vi "RegisterGUIObjectToResize.vi"(5 "Resize Object?":bool=TRUE, 8 "error in (no error)":errorcluster, 9 "Behaviour":T1 {"Adjust" items=["Height", "Width", "Both"]}, 10 "Any Control reference":refnum<vi>, 11 "PentaPanesGUI in":refnum<class "PentaPanes.lvclass">) -> (0 "error out":errorcluster, 1 "Class Name":string, 2 "OwningPane":refnum<vi>, 3 "PentaPanesGUI out":refnum<class "PentaPanes.lvclass">)   [LabVIEW 2022 SP3, in "PentaPanesLibrary.lvlib" / "PentaPanes.lvclass"]
doc: "This VI registers a reference of a control object (String, Array, XYGraph etc.) and it's resize behaviour. \nfor use with future resizing methods. \n \nPentaPanesGUI in - PentaPanesObject in\nPenraPanesGUI out - PentaPanesObject out\nAny control reference - The reference of the control object registering to be scaled\nBehaviour - resizing Behaviour Cluster\n Adjust - Adjust Height (0), Width (1) or Both (2)\n Borders - Spaces around the object in the pane. \n Borders in Percent - Borders units are in percent of pane (T) or Pixels (F)\n Minimal - Minimum size control can be set to. \n Invisible - Set object to invisible (T) or Visible (F) \n -- note - objects don't get resized while invisible is on. \n Force Aspect Ratio - Forces draw area to fit graph axes (T)\nResize Object? - If true resizes the objects in the Pane that owns the object.\nOwning Pane - outputs the reference of the pane that the object belongs to.\nClass Name - outputs the name of the class the of the registering control"
uses:
  PentaPanes.lvclass
  ResizeBehaviourCluster.ctl
  BordersCluster.ctl
  <vilib>/Utility/miscctls.llb/LVBoundsTypeDef.ctl
  ResizableObject.ctl
  PentaPanes.lvclass/PentaPanes.ctl
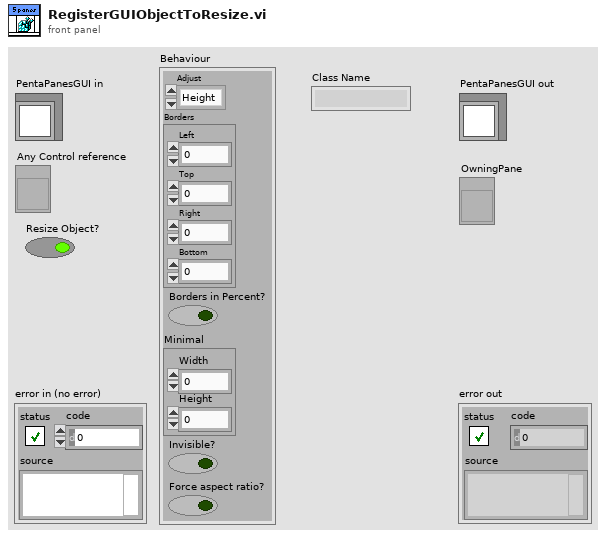
[diagram p1: front panel]
types:
  T1 = typedef "PentaPanesLibrary.lvlib/PentaPanes.lvclass/ResizeBehaviourCluster.ctl" = cluster{"Adjust":u16, "Borders":T2, "Borders in Percent?":bool, "Minimal":T3, "Invisible?":bool, "Force aspect ratio?":bool}
  T2 = typedef "PentaPanesLibrary.lvlib/PentaPanes.lvclass/BordersCluster.ctl" = cluster{"Left":i32, "Top":i32, "Right":i32, "Bottom":i32}
  T3 = typedef "LVBoundsTypeDef.ctl" = cluster{"Width":i32, "Height":i32}
  T4 = typedef "PentaPanesLibrary.lvlib/PentaPanes.lvclass/ResizableObject.ctl" = cluster{"generic class reference":refnum<vi>, "Label out":string, "Adjust":u16, "Borders":T2, "Minimal":T3, "Class Name out":string, "Class ID out":u32, "Owning Pane out":refnum<vi>, "Borders in Percent(T) or Pixels (F)":bool, "Invisible?":bool, "Force Aspect Ratio?":bool}
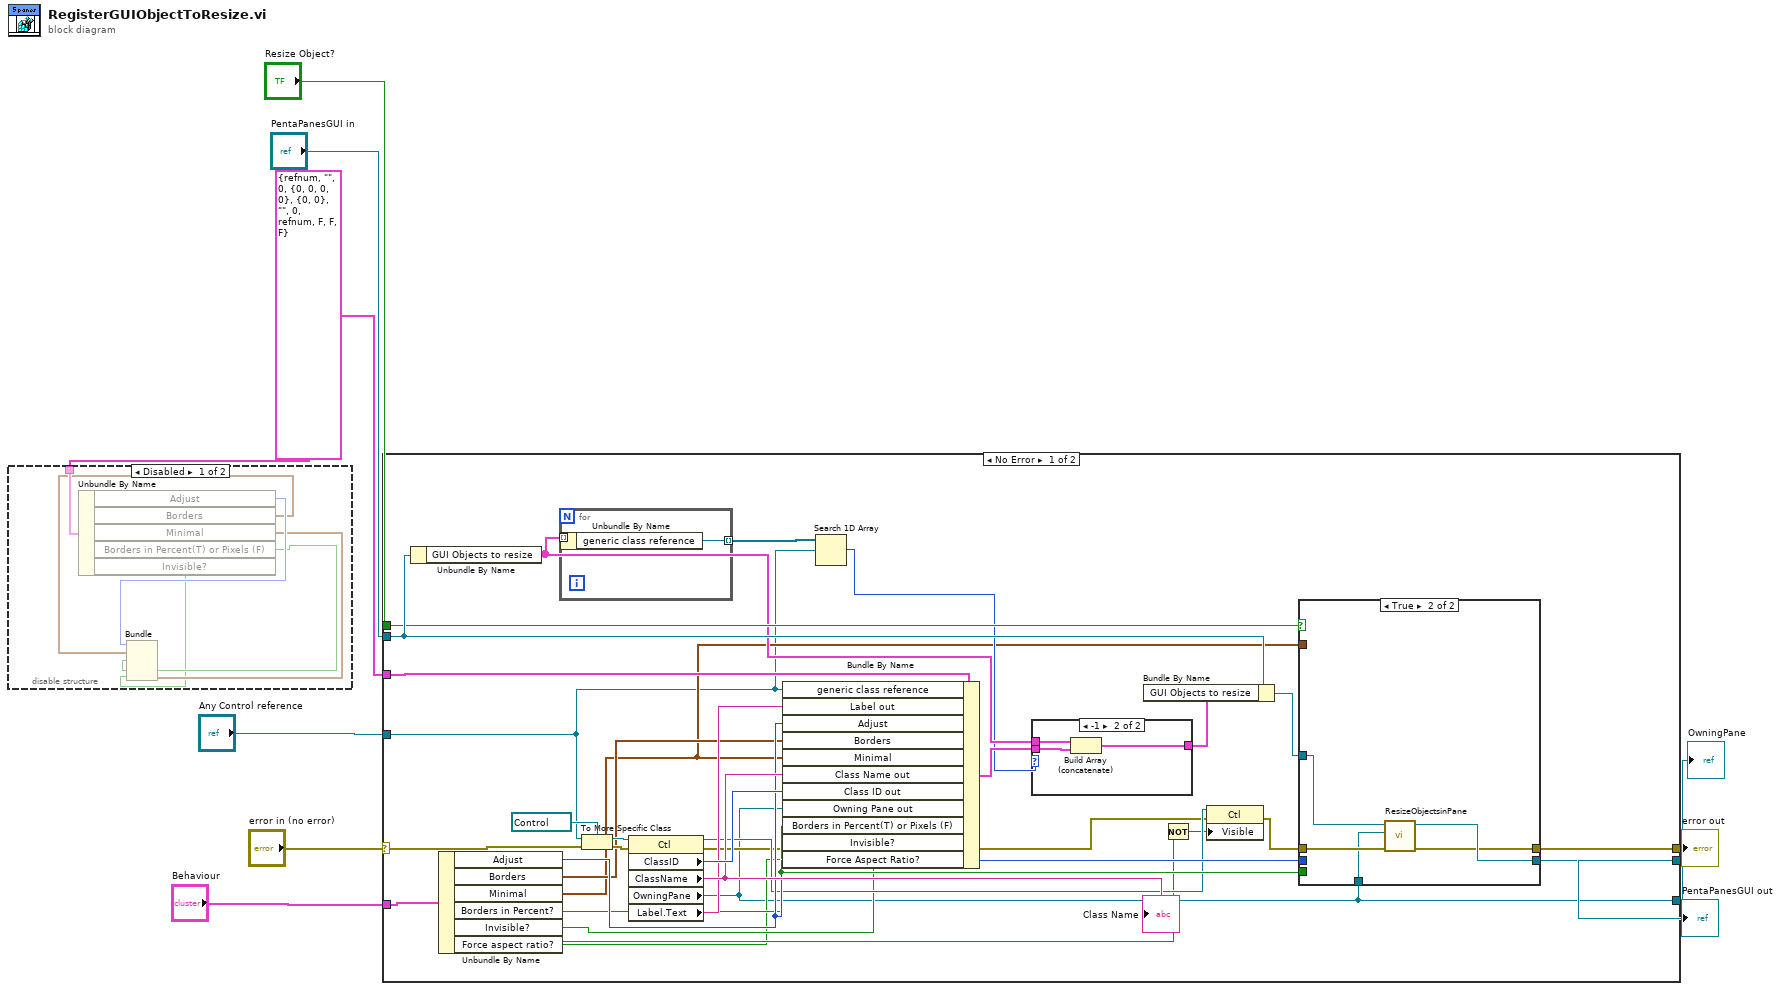
[diagram p0: block diagram]
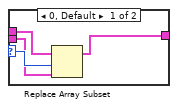
[diagram p3: hidden frame]
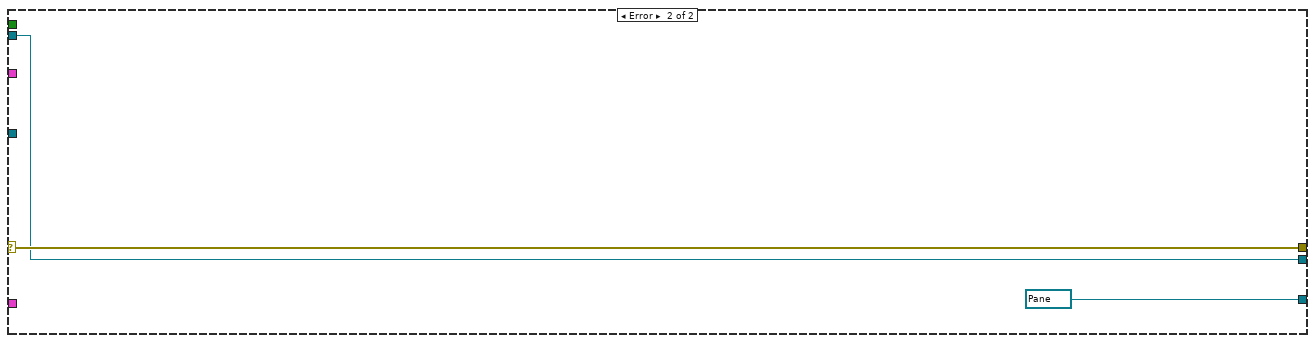
[diagram p5: hidden frame]
diagram:
  w2 = T4 {"generic class reference"=refnum, "Label out"="", "Adjust"=0, "Borders"={"Left"=0, "Top"=0, "Right"=0, "Bottom"=0}, "Minimal"={"Width"=0, "Height"=0}, "Class Name out"="", "Class ID out"=0, "Owning Pane out"=refnum, "Borders in Percent(T) or Pixels (F)"=FALSE, "Invisible?"=FALSE, "Force Aspect Ratio?"=FALSE}
  n1 = disable-structure shown="Disabled" {
    disable-tunnel: w2 -> [w15 _]
    frame Disabled {
      n2 = Unbundle By Name(w15) -> ("Adjust"=w14:u16, "Borders"=w13:T2, "Minimal"=w11:T3, "Borders in Percent(T) or Pixels (F)"=w12:bool, "Invisible?"=w10:bool)
      n3 = Bundle("Adjust"=w14, "Borders"=w13, "Borders in Percent(T) or Pixels (F)"=w12, "Minimal"=w11, "Invisible?"=w10) -> ()  [unwired: 1 in, 1 out]
    }
    frame Enabled {
    }
  }
  n4 = case shown="No Error" "error in (no error)" {
    selector: "error in (no error)" -> [w39 w65]
    tunnel: [w19 w65] -> w8
    tunnel: [w35 w64] -> w6
    tunnel: "PentaPanesGUI in" -> [w46 w64]
    tunnel: w2 -> [w43 _]
    tunnel: "Any Control reference" -> [w24 _]
    tunnel: "Resize Object?" -> [w34 _]
    tunnel: [w16 refnum<vi> refnum ("OwningPane")] -> w3
    tunnel: "Behaviour" -> [w29 _]
    frame No Error {
      n5 = Unbundle By Name(w46) -> ("GUI Objects to resize"=w32:T4[])
      n6 = Unbundle By Name(w29) -> ("Adjust"=w28:u16, "Borders"=w27:T2, "Minimal"=w26:T3, "Borders in Percent?"=w25:bool, "Invisible?"=w21:bool, "Force aspect ratio?"=w20:bool)
      n7 = for {
        tunnel: w32 -> [w55] mode=indexing
        tunnel: [w54] -> w31 mode=indexing
        n8 = Unbundle By Name(w55) -> ("generic class reference"=w54:refnum<vi>)
      }
      n9 = To More Specific Class(target class=refnum<vi> refnum ("generic class reference"), reference=w24, error in=w39) -> (specific class reference=w41:refnum<vi>, error out=w40:errorcluster)
      n10 = property class="Ctl"(reference=w41, error in=w40) -> (reference out=w23:refnum<vi>, error out=w18:errorcluster, "ClassID"=w38:u32, "ClassName"=w37:string, "OwningPane"=w16:refnum<vi>, "Label.Text"=w33:string)
      "Class Name" <- w37
      n11 = Bundle By Name(cluster=w43, "generic class reference"=w24, "Label out"=w33, "Adjust"=w28, "Borders"=w27, "Minimal"=w26, "Class Name out"=w37, "Class ID out"=w38, "Owning Pane out"=w16, "Borders in Percent(T) or Pixels (F)"=w25, "Invisible?"=w21, "Force Aspect Ratio?"=w20) -> (w44:T4)
      n12 = Search 1D Array(1D array=w31, element=w24) -> (index of element=w30:i32)  [unwired: 1 in]
      n13 = case shown="-1" w30 {
        selector: w30 -> [w49 _]
        tunnel: [w47 w53] -> w45
        tunnel: w44 -> [w48 w52]
        tunnel: w32 -> [w50 w51]
        frame 0, Default {
          n14 = Replace Array Subset "Replace Array Subset"(array=w50, new element=w48, index=w49) -> (w47:T4[])
        }
        frame -1 {
          n15 = Build Array (concatenate)(w51, w52) -> (w53:T4[])
        }
      }
      n16 = Bundle By Name(cluster=w46, "GUI Objects to resize"=w45) -> (w36:refnum<class "PentaPanes.lvclass">)
      n17 = Not(x=w21) -> (.not. x?=w22:bool)
      n18 = property class="Ctl"(reference=w23, error in=w18, "Visible"=w22) -> (error out=w17:errorcluster)  [unwired: 1 out]
      n19 = case shown="True" w34 {
        tunnel: w36 -> [w57 w59]
        tunnel: [w57 w62] -> w35
        tunnel: w26 -> [_ _]
        tunnel: w17 -> [w56 w61]
        tunnel: [w56 w60] -> w19
        tunnel: w28 -> [_ _]
        tunnel: w25 -> [_ _]
        tunnel: w16 -> [_ w58]
        frame False {
        }
        frame True {
          n20 = call-dynamic "ResizeObjectsinPane.vi"("error in (no error)"=w61, "PaneRef"=w58, "PentaPanesGUI in"=w59) -> ("error out"=w60:errorcluster, "PentaPanesGUI out"=w62:refnum<class "PentaPanes.lvclass">)  [unwired: 7 in]
        }
      }
    }
    frame Error {
    }
  }
  "error out" <- w8
  "PentaPanesGUI out" <- w6
  "OwningPane" <- w3
